vi "Read PressureDisplay Setup.vi"(11 "VacuumLines in":refnum<class "VacuumLines.lvclass">) -> (2 "PressureDisplay Setup":T1[](array[typedef]) {"Threshold" format="%#.1e"}, 3 "VacuumLines out":refnum<class "VacuumLines.lvclass">)   [LabVIEW 2016, in "Hardware.lvlib" / "VacuumLine.lvlib" / "VacuumLines.lvclass"]
uses:
  <userlib>/Common Components/Hardware/Abstract System/VacuumLine/VacuumLines/VacuumLines.lvclass
  <userlib>/Common Components/Hardware/Abstract System/VacuumLine/VacuumLines/Gauge Param.ctl
  <userlib>/Common Components/Hardware/Abstract System/VacuumLine/VacuumLines/VacuumLines.lvclass/VacuumLines.ctl
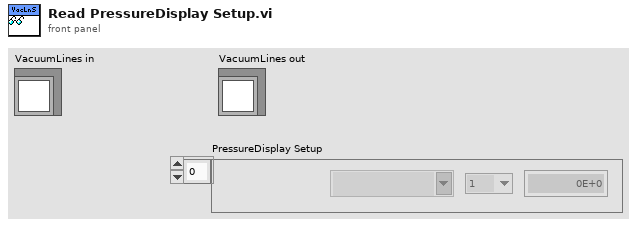
[diagram p1: front panel]
types:
  T1 = typedef "Hardware.lvlib/VacuumLine.lvlib/VacuumLines.lvclass/Gauge Param.ctl" = cluster{"label":string, "Gauge Controller":string, "Channel":enum16{"1", "2", "3", "4", "5", "6", "7", "8"}, "Threshold":dbl}
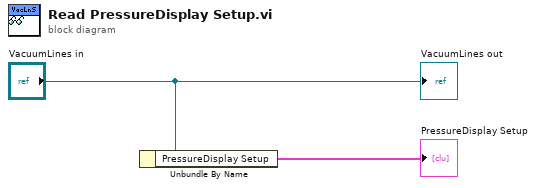
[diagram p0: block diagram]
diagram:
  n1 = Unbundle By Name("VacuumLines in") -> ("PressureDisplay Setup"=→"PressureDisplay Setup":T1[])
  "VacuumLines out" <- "VacuumLines in"
